vi "Pulser Protect Tripped Status.vi"(8 "error in (no error)":errorcluster, 10 "Source Measure Unit Channel (0: Channel A)":i32(ring) items=["Channel A", "Channel B"], 11 "VISA resource name":refnum<visa-resource-name>) -> (0 "error out":errorcluster, 2 "Tripped Status":bool, 3 "VISA resource name out":refnum<visa-resource-name>)   [LabVIEW 2019, in "Keithley 2600 Series.lvlib"]
doc: "Returns the voltage protection status; indicates if either protection limit is exceeded."
uses:
  Keithley 2600 Series.lvlib
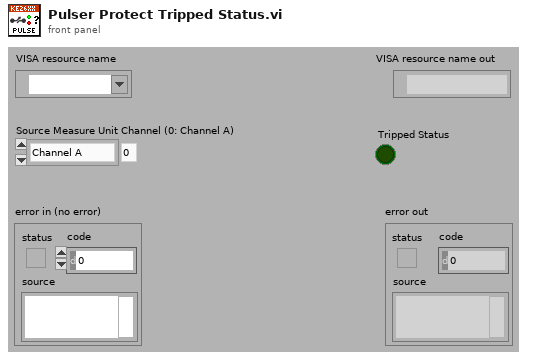
[diagram p1: front panel]
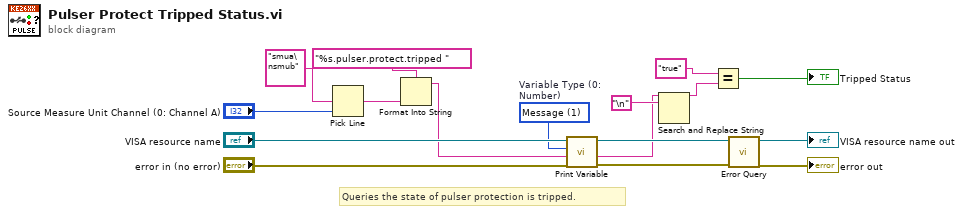
[diagram p0: block diagram]
diagram:
  w8 = 1 items=["Number", "Message"]  # Variable Type (0: Number)
  # "Queries the state of pulser protection is tripped."
  n1 = Pick Line(multi-line string="smua\nsmub", line index="Source Measure Unit Channel (0: Channel A)") -> (output string=w10:string)  [unwired: 1 in]
  n2 = Format Into String(format string="%s.pulser.protect.tripped ", w10) -> (resulting string=w4:string)  [unwired: 2 in, 1 out]
  n3 = call "Print Variable.vi"("error in (no error)"="error in (no error)", "Variable Name"=w4, "Variable Type (0: Number)"=w8, "VISA resource name"="VISA resource name") -> ("error out"=w5:errorcluster, "Message"=w1:string, "VISA resource name out"=w7:refnum<visa-resource-name>)  [unwired: 4 in, 1 out]
  n4 = Search and Replace String(input string=w1, search string="\n") -> (result string=w3:string)  [unwired: 6 in, 3 out]
  n5 = Equal?(x="true", y=w3) -> (x = y?=→"Tripped Status":bool)
  n6 = call "Error Query.vi"("error in (no error)"=w5, "VISA resource name"=w7) -> ("error out"=→"error out":errorcluster, "VISA resource name out"=→"VISA resource name out":refnum<visa-resource-name>)  [unwired: 6 in, 2 out]
